vi "Open Excel File.vi"(8 "error in (no error)":errorcluster, 10 "File Name":path) -> (0 "error out":errorcluster, 3 "IWorkbook Reference Out":refnum<k24>)   [LabVIEW 2014]
uses:
  C:/Users/LENOVO/Desktop/CodeSpace GUI/LVExcel/Resources/net40/NPOI.dll
  Resources/net40/NPOI.dll
  C:/Users/LENOVO/Desktop/CodeSpace GUI/LVExcel/Resources/net40/NPOI.OOXML.dll
  Resources/net40/NPOI.OOXML.dll
  <vilib>/Utility/error.llb/Error Cluster From Error Code.vi
  <vilib>/ErrorRing/Error Ring.xnode
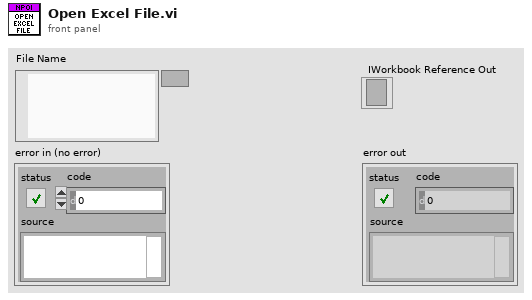
[diagram p1: front panel]
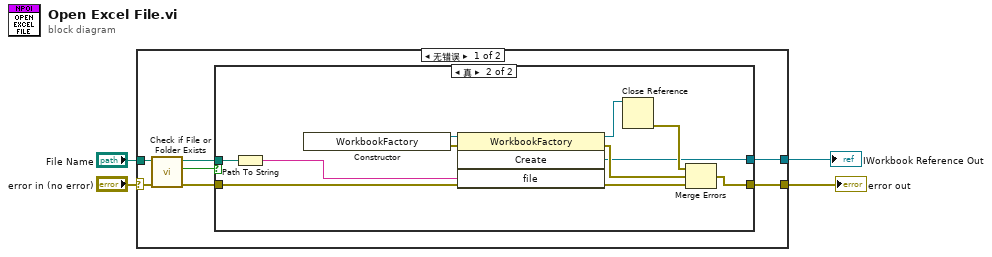
[diagram p0: block diagram]
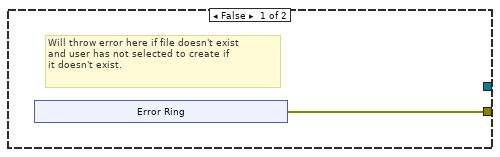
[diagram p2: hidden frame]
diagram:
  n1 = case shown="无错误" "error in (no error)" {
    selector: "error in (no error)" -> [w5 w27]
    tunnel: [w11 w27] -> w4
    tunnel: "File Name" -> [w10 _]
    tunnel: [w6 _] -> w2
    frame No Error {
      n2 = call <vilib>:"Check if File or Folder Exists.vi"("error in (no error)"=w5, "path"=w10) -> ("error out"=w8:errorcluster, "file or folder exists?"=w7:bool, "dup path"=w9:path)  [unwired: 7 in]
      n3 = case shown="真" w7 {
        tunnel: [w12 w19] -> w11
        tunnel: w8 -> [_ w18]
        tunnel: w9 -> [_ w26]
        tunnel: [_ w20] -> w6
        frame False {
          # "Will throw error here if file doesn't exist\nand user has not selected to create if\nit doesn't exist."
          n4 = xnode "Error Ring"() -> ("错误输出"=w12:errorcluster)
        }
        frame True {
          n5 = Path To String(path=w26) -> (string=w17:string)
          n6 = constructor class="WorkbookFactory"() -> (reference out=w21:refnum<k24>, error out=w22:errorcluster)  [unwired: 3 in, 1 out]
          n7 = invoke class="WorkbookFactory" method="Create"(reference=w21, error in=w22, "file"=w17) -> (reference out=w23:refnum<k24>, error out=w24:errorcluster, "Create"=w20:refnum<k24>)  [unwired: 1 in, 1 out]
          n8 = Close Reference(reference=w23) -> (error out=w25:errorcluster)  [unwired: 1 in]
          n9 = Merge Errors(w25, w24, w18) -> (w19:errorcluster)
        }
      }
    }
    frame Error {
    }
  }
  "IWorkbook Reference Out" <- w2
  "error out" <- w4
